vi "REPETICIONES_CICLOS.vi"(8 "error in (no error)":errorcluster, 10 "Secuencia":string[](array[string])=["Posicion jeringa: Setpoint: 10.000 mm", "Repetir:  3  veces", "Presión línea: Setpoint: 100.0 mmHg, Error:  2.0 mmHg, Timeout:  1.0 min", "Tiempo de medida: 2.0 min:", "Presión línea: Setpoint: 200.0 mmHg, Error:  2.0 mmHg, Timeout:  1.0 min", "Tiempo de medida: 2.0 min:", "Fin repeticiones", "Posicion jeringa: Setpoint: 10.000 mm", "Repetir:  3  veces", "Presión línea: Setpoint: 100.0 mmHg, Error:  2.0 mmHg, Timeout:  1.0 min", "Tiempo de medida: 2.0 min:", "Presión línea: Setpoint: 200.0 mmHg, Error:  2.0 mmHg, Timeout:  1.0 min", "Tiempo de medida: 2.0 min:", "Fin repeticiones"]) -> (0 "error out":errorcluster, 1 "Secuciclos":string[](array[string]))   [LabVIEW 2017]
panel:
  out "Array f":i32[](array[numeric])
  out "Array i":i32[](array[numeric])
  out "Array rep":i32[](array[numeric])
  out "Repeticiones":i32
  out "Indices StopRep":i32
  out "Indices StartRep":i32
  # "Programador de comandos"
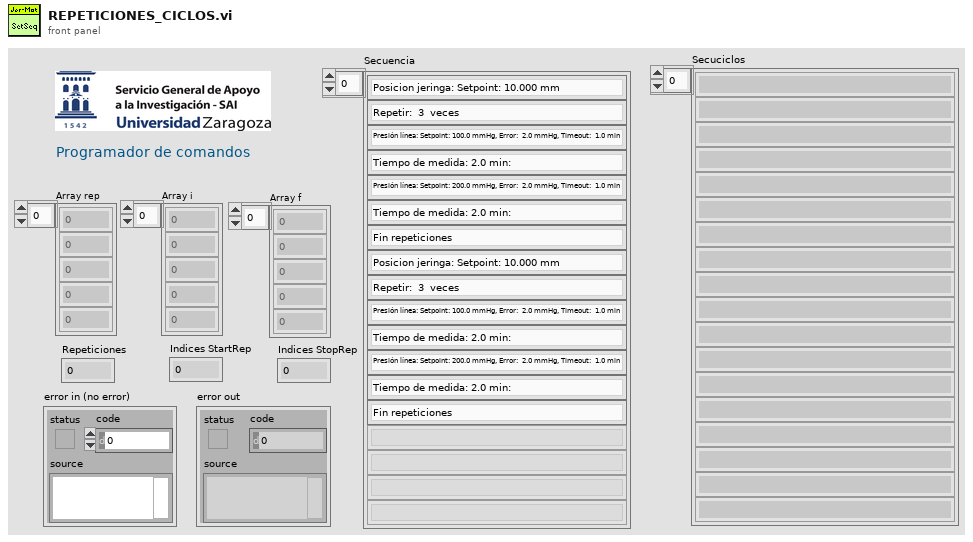
[diagram p1: front panel]
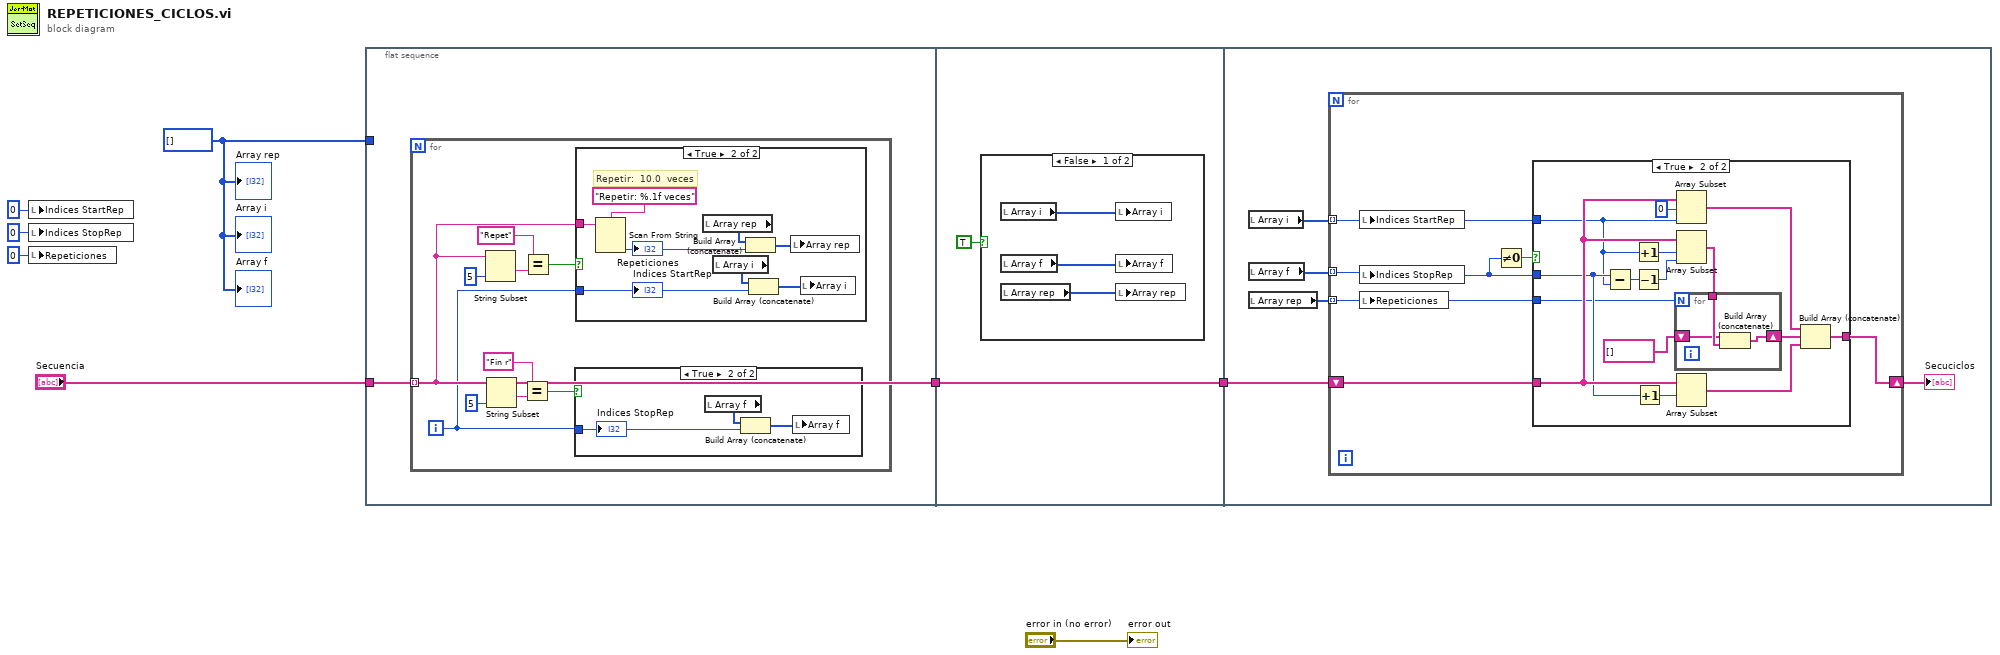
[diagram p0: block diagram]
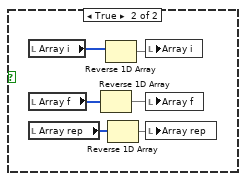
[diagram p4: hidden frame]
diagram:
  w3 = i32[] [] ("Array rep")
  n1 = local write "Indices StartRep"(0 ("Indices StartRep")) -> ()
  n2 = local write "Indices StopRep"(0 ("Indices StopRep")) -> ()
  n3 = local write "Repeticiones"(0 ("Repeticiones")) -> ()
  n4 = flat-sequence {
    tunnel: "Secuencia" -> [w9]
    tunnel: [w9] -> w2
    tunnel: w3 -> [_]
    tunnel: w2 -> [w32]
    tunnel: [w32] -> w1
    tunnel: w1 -> [w46]
    frame #0 {
      n5 = for {
        tunnel: w9 -> [w12] mode=indexing
        i -> [w11]
        n6 = String Subset(string=w12, length (rest)=5 ("length (rest)")) -> (substring=w18:string)  [unwired: 1 in]
        n7 = String Subset(string=w12, length (rest)=5 ("length (rest)")) -> (substring=w14:string)  [unwired: 1 in]
        n8 = Equal?(x="Fin r" ("input 1"), y=w14) -> (x = y?=w10:bool)
        n9 = Equal?(x="Repet" ("input 1"), y=w18) -> (x = y?=w16:bool)
        n10 = case shown="True" w10 {
          tunnel: w11 -> [_ w20]
          frame False {
          }
          frame True {
            n11 = local read "Array f"() -> (w22:i32[])
            n12 = Build Array (concatenate)(w22, w20) -> (w21:i32[])
            n13 = local write "Array f"(w21) -> ()
            "Indices StopRep" <- w20
          }
        }
        n14 = case shown="True" w16 {
          tunnel: w11 -> [_ w24]
          tunnel: w12 -> [_ w29]
          frame False {
          }
          frame True {
            # "Repetir:  10.0  veces"
            n15 = Scan From String(format string="Repetir: %.1f veces", input string=w29) -> (output 1=w23:i32)  [unwired: 3 in, 3 out]
            "Repeticiones" <- w23
            n16 = local read "Array rep"() -> (w27:i32[])
            n17 = local read "Array i"() -> (w26:i32[])
            n18 = Build Array (concatenate)(w27, w23) -> (w28:i32[])
            n19 = Build Array (concatenate)(w26, w24) -> (w25:i32[])
            n20 = local write "Array rep"(w28) -> ()
            n21 = local write "Array i"(w25) -> ()
            "Indices StartRep" <- w24
          }
        }
      }
    }
    frame #1 {
      n22 = case shown="False" TRUE {
        frame False {
          n23 = local read "Array i"() -> (w35:i32[])
          n24 = local read "Array f"() -> (w34:i32[])
          n25 = local read "Array rep"() -> (w33:i32[])
          n26 = local write "Array i"(w35) -> ()
          n27 = local write "Array f"(w34) -> ()
          n28 = local write "Array rep"(w33) -> ()
        }
        frame True {
          n29 = local read "Array i"() -> (w37:i32[])
          n30 = local read "Array f"() -> (w39:i32[])
          n31 = local read "Array rep"() -> (w41:i32[])
          n32 = Reverse 1D Array(array=w39) -> (reversed array=w38:i32[])
          n33 = Reverse 1D Array(array=w37) -> (reversed array=w36:i32[])
          n34 = Reverse 1D Array(array=w41) -> (reversed array=w40:i32[])
          n35 = local write "Array i"(w36) -> ()
          n36 = local write "Array f"(w38) -> ()
          n37 = local write "Array rep"(w40) -> ()
        }
      }
    }
    frame #2 {
      n38 = local read "Array i"() -> (w43:i32[])
      n39 = local read "Array f"() -> (w45:i32[])
      n40 = local read "Array rep"() -> (w42:i32[])
      n41 = for {
        tunnel: w45 -> [w47] mode=indexing
        shift-right: [w50] -> w44
        shift-left: w46 -> [w52]
        tunnel: w43 -> [w49] mode=indexing
        tunnel: w42 -> [w48] mode=indexing
        n42 = local write "Indices StartRep"(w49) -> ()
        n43 = local write "Indices StopRep"(w47) -> ()
        n44 = local write "Repeticiones"(w48) -> ()
        n45 = Not Equal To 0?(x=w47) -> (x != 0?=w51:bool)
        n46 = case shown="True" w51 {
          tunnel: [w53 w68] -> w50
          tunnel: w52 -> [w53 w57]
          tunnel: w47 -> [_ w56]
          tunnel: w49 -> [_ w55]
          tunnel: w48 -> [_ w54]
          frame False {
          }
          frame True {
            n47 = Subtract(x=w56, y=w55) -> (x-y=w59:i32)
            n48 = Increment(x=w55) -> (x+1=w63:i32)
            n49 = Decrement(x=w59) -> (x-1=w62:i32)
            n50 = Increment(x=w56) -> (x+1=w64:i32)
            n51 = Array Subset(array=w57, index=0, length=w55) -> (w67:string[])
            n52 = Array Subset(array=w57, index=w63, length=w62) -> (w60:string[])
            n53 = for {
              N: w54 -> [_]
              tunnel: w60 -> [w71]
              shift-right: [w69] -> w58
              shift-left: string[] [] ("element") -> [w70]
              n54 = Build Array (concatenate)(w70, w71) -> (w69:string[])
            }
            n55 = Array Subset(array=w57, index=w64) -> (w65:string[])  [unwired: 1 in]
            n56 = Build Array (concatenate)(w67, w58, w65) -> (w68:string[])
          }
        }
      }
      "Secuciclos" <- w44
    }
  }
  "error out" <- "error in (no error)"
  "Array rep" <- w3
  "Array i" <- w3
  "Array f" <- w3
